vi "Simulate Rop Graph.vi"() -> ()   [LabVIEW 2020, in "AoC 2022.lvlib"]
uses:
  AoC 2022.lvlib
panel:
  in  "Puzzle Input":string="L 1\nD 2\nU 1\nL 1\nR 2\nL 2\nU 1\nD 2\nR 2\nL 2\nU 1\nD 2\nR 1\nD 2\nL 2\nD 1\nL 2\nR 1\nU 2\nR 2\nU 2\nL 2\nU 1\nL 2\nR 1\nD 1\nR 1\nL 1\nR 1\nL 1\nR 1\nU 1\nR 1\nL 1\nD 2\nL 2\nD 2\nL 1\nR 1\nD 1\nR 1\nD 2\nL 1\nD 2\nL 1\nR 2\nD 2\nR 2\nU 1\nR 1\nU 2\nR 1\nU 2\nR 1\nD 2\nL 1\nD 2\nU 1\nR 2\nD 2\nL 1\nU 2\nR 2\nL 2\nD 2\nL 2\nD 2\nR 1\nU 2\nL 2\nU 1\nR 1\nD 1\nL 1\nD 1\nU 1\nD 2\nL 1\nR 1\nD 1\nR 1\nL 2\nR 1\nL 1\nU 2\nD 2\nU 1\nL 1\nU 2\nR 1\nD 2\nU 1\nD 1\nL 1\nD 2\nU 2\nD 1\nU 2\nR 2\nL 2\nD 1\nR 2\nD 1\nL 2\nD 2\nL 2\nR 1\nL 1\nR 2\nL 2\nR 2\nU 1\nR 1\nU 3\nD 2\nU 3\nL 1\nR 1\nU 3\nD 1\nL 1\nR 3\nD 2\nL 3\nR 3\nD 2\nR 2\nU 3\nR 3\nU 3\nR 2\nU 3\nD 2\nL 3\nU 3\nR 1\nU 1\nR 3\nU 2\nL 1\nR 1\nU 1\nL 3\nR 3\nU 3\nD 2\nU 1\nL 1\nD 3\nR 3\nU 2\nL 1\nR 3\nL 3\nD 3\nU 3\nR 2\nL 1\nU 1\nL 3\nR 3\nU 1\nR 3\nL 2\nR 2\nD 3\nU 1\nD 3\nU 3\nR 3\nD 2\nL 2\nU 2\nD 3\nL 3\nU 3\nR 3\nD 2\nR 3\nU 1\nD 1\nU 2\nR 1\nD 3\nR 1\nL 2\nU 3\nD 1\nL 1\nD 3\nU 2\nL 3\nR 3\nL 1\nD 2\nL 3\nU 3\nL 1\nD 2\nL 1\nD 1\nL 2\nU 2\nD 2\nU 2\nL 2\nD 3\nL 3\nD 3\nR 3\nU 1\nR 3\nU 1\nR 3\nD 3\nU 2\nD 1\nR 2\nL 2\nR 2\nD 2\nR 2\nD 1\nR 3\nD 1\nU 2\nL 4\nD 1\nL 2\nR 1\nU 1\nD 3\nU 4\nD 2\nL 3\nR 2\nD 3\nR 4\nU 1\nD 1\nU 1\nL 3\nU 1\nD 3\nR 3\nD 3\nR 1\nU 4\nR 1\nU 1\nR 2\nL 4\nU 3\nD 2\nR 2\nD 1\nU 2\nL 3\nD 4\nU 4\nD 4\nU 4\nL 3\nU 3\nD 3\nR 3\nL 4\nR 3\nD 2\nL 2\nR 1\nD 1\nL 4\nR 3\nD 2\nU 1\nL 2\nR 1\nU 2\nL 4\nR 4\nL 3\nU 4\nD 2\nU 4\nD 4\nL 1\nU 4\nL 3\nU 2\nD 2\nR 2\nD 3\nR 4\nD 1\nU 4\nD 1\nU 1\nD 3\nL 3\nD 2\nR 4\nD 4\nL 2\nU 2\nL 3\nR 4\nL 2\nR 2\nD 3\nL 2\nD 4\nU 3\nD 4\nL 3\nR 2\nU 3\nD 4\nR 2\nU 3\nR 1\nD 1\nR 1\nD 2\nR 3\nD 4\nL 1\nU 3\nL 3\nU 4\nR 1\nU 3\nL 4\nD 5\nR 2\nD 2\nU 2\nD 1\nR 4\nD 1\nL 4\nD 4\nL 1\nR 1\nD 4\nU 4\nL 1\nD 4\nL 4\nU 5\nR 4\nD 4\nR 5\nU 3\nL 5\nU 1\nR 4\nL 1\nR 3\nL 2\nD 5\nR 1\nD 4\nR 2\nU 5\nL 3\nR 5\nU 4\nR 1\nD 4\nU 3\nR 3\nL 3\nR 3\nL 3\nU 2\nD 4\nU 2\nL 3\nD 2\nR 3\nU 3\nD 2\nU 1\nR 5\nL 4\nR 4\nL 4\nD 3\nR 3\nU 2\nR 1\nD 3\nU 3\nD 2\nL 1\nD 2\nU 1\nL 3\nU 5\nL 1\nD 1\nU 5\nD 3\nU 4\nD 4\nL 5\nR 3\nD 4\nR 2\nL 1\nD 1\nL 3\nU 3\nR 1\nL 2\nD 4\nL 5\nU 1\nL 4\nR 4\nU 2\nD 1\nR 5\nD 3\nU 2\nD 3\nU 4\nD 4\nU 1\nL 2\nD 4\nL 3\nU 4\nL 1\nR 1\nL 2\nR 3\nL 2\nU 1\nD 2\nU 5\nR 2\nD 4\nU 1\nD 4\nU 4\nD 5\nL 6\nD 3\nU 2\nD 1\nL 3\nU 4\nR 4\nD 4\nR 3\nL 4\nU 6\nD 1\nU 4\nR 2\nL 1\nD 2\nU 4\nD 5\nU 3\nD 6\nL 1\nU 3\nL 1\nU 1\nD 6\nL 3\nU 6\nL 3\nD 6\nL 1\nD 6\nU 2\nD 5\nU 2\nL 5\nD 3\nU 2\nD 1\nU 6\nL 1\nD 4\nL 6\nR 3\nD 3\nL 3\nD 2\nR 3\nD 5\nR 3\nD 2\nL 1\nR 4\nL 6\nD 4\nR 4\nU 1\nR 6\nD 3\nU 1\nR 1\nD 1\nL 3\nD 1\nR 3\nU 5\nL 5\nD 2\nL 3\nD 2\nL 5\nU 3\nL 1\nU 5\nL 3\nD 4\nU 5\nD 1\nL 6\nD 1\nR 6\nU 4\nR 1\nD 1\nL 2\nU 5\nR 2\nU 6\nL 5\nU 5\nL 6\nU 6\nD 3\nL 1\nR 3\nL 3\nU 4\nR 5\nL 6\nD 5\nL 4\nR 6\nL 6\nR 5\nD 2\nR 4\nL 2\nU 1\nL 3\nU 6\nL 4\nD 6\nU 6\nD 4\nL 2\nR 7\nU 4\nR 1\nL 5\nD 2\nR 3\nU 4\nL 5\nU 7\nL 2\nR 1\nU 4\nL 2\nR 5\nL 6\nD 5\nL 4\nU 5\nL 7\nU 1\nL 5\nU 1\nL 5\nD 3\nU 3\nR 7\nU 7\nR 7\nL 6\nD 4\nU 7\nR 2\nD 3\nR 3\nU 4\nD 4\nU 5\nD 6\nL 5\nR 6\nU 4\nR 6\nD 1\nR 4\nU 1\nD 1\nR 1\nL 4\nU 5\nL 3\nD 5\nL 5\nD 3\nU 2\nR 5\nD 7\nU 7\nD 1\nU 5\nR 6\nU 4\nR 6\nL 7\nU 5\nR 1\nL 1\nU 1\nR 1\nD 7\nL 2\nU 5\nR 4\nU 2\nD 6\nU 6\nL 7\nU 3\nD 2\nL 3\nR 3\nU 2\nL 1\nR 2\nL 5\nD 6\nR 2\nU 6\nL 1\nD 7\nR 4\nD 3\nL 2\nU 5\nR 4\nL 2\nR 5\nD 1\nU 1\nR 6\nD 5\nU 6\nR 2\nU 2\nL 2\nU 6\nL 5\nU 1\nL 1\nD 7\nR 6\nU 5\nD 3\nL 5\nR 3\nD 3\nU 2\nD 7\nU 7\nL 1\nD 5\nL 5\nU 4\nL 5\nD 1\nU 6\nD 5\nL 7\nD 8\nU 8\nR 6\nU 5\nD 8\nU 1\nR 2\nU 6\nD 6\nL 4\nD 2\nR 3\nU 7\nR 4\nU 4\nR 5\nU 6\nR 1\nU 4\nR 1\nU 4\nD 5\nU 3\nL 7\nU 8\nR 1\nD 1\nU 8\nL 8\nU 3\nL 1\nD 4\nR 2\nD 4\nU 2\nL 4\nD 8\nR 7\nD 5\nU 4\nL 5\nU 5\nD 8\nR 8\nU 3\nR 8\nL 4\nU 5\nR 6\nU 7\nD 3\nL 1\nU 5\nD 2\nR 5\nU 4\nD 8\nL 4\nR 1\nD 6\nR 1\nL 6\nD 6\nL 7\nD 4\nL 4\nD 8\nR 8\nD 7\nL 6\nR 1\nD 4\nL 5\nD 2\nU 3\nD 2\nU 6\nR 1\nU 7\nD 7\nR 2\nU 7\nD 5\nL 6\nU 1\nL 8\nU 1\nL 1\nR 9\nD 1\nU 6\nD 5\nL 1\nR 9\nD 2\nL 2\nD 6\nU 6\nD 7\nL 3\nR 5\nL 6\nU 5\nR 1\nU 1\nR 3\nL 9\nU 6\nL 6\nU 2\nD 6\nR 9\nU 4\nD 3\nL 8\nU 5\nD 7\nL 1\nU 7\nR 1\nL 6\nD 8\nL 5\nR 7\nL 2\nR 6\nL 5\nD 3\nL 8\nD 7\nU 8\nR 6\nL 6\nD 7\nU 8\nD 1\nU 2\nD 5\nU 7\nD 8\nL 1\nD 1\nL 1\nU 1\nR 3\nL 5\nR 9\nD 2\nL 8\nR 6\nD 6\nU 1\nR 7\nL 4\nU 4\nD 1\nL 5\nU 2\nR 9\nD 7\nU 8\nL 8\nR 4\nD 1\nL 1\nU 7\nR 8\nL 3\nD 2\nU 8\nR 1\nD 5\nL 1\nR 7\nD 6\nR 2\nU 9\nD 2\nL 5\nU 4\nD 9\nL 7\nD 9\nL 2\nU 9\nD 5\nL 7\nD 6\nU 5\nD 9\nR 3\nU 8\nL 7\nU 1\nL 3\nU 3\nD 1\nL 6\nR 9\nU 2\nL 7\nR 9\nU 5\nR 2\nL 3\nR 4\nD 9\nL 4\nR 9\nU 4\nL 10\nR 9\nD 9\nU 10\nL 2\nR 4\nU 4\nR 9\nD 2\nR 1\nL 4\nR 7\nD 3\nL 6\nU 1\nL 9\nD 6\nU 10\nD 1\nR 10\nD 9\nL 6\nD 10\nU 3\nR 10\nL 8\nU 9\nD 1\nL 1\nD 10\nL 1\nD 5\nL 9\nU 3\nL 4\nU 4\nD 1\nU 3\nR 7\nL 3\nR 3\nL 3\nR 8\nD 9\nR 4\nL 6\nD 7\nR 10\nU 6\nR 2\nD 2\nL 3\nR 9\nD 9\nU 7\nD 2\nR 6\nU 10\nR 8\nU 5\nR 5\nU 10\nR 6\nU 7\nL 7\nU 7\nD 4\nL 9\nU 2\nR 7\nL 8\nR 4\nL 1\nU 9\nR 8\nD 4\nR 5\nD 4\nL 1\nD 10\nR 8\nD 10\nU 9\nD 3\nR 1\nU 10\nR 1\nD 10\nR 1\nL 6\nD 3\nU 8\nR 4\nU 9\nD 8\nU 3\nD 2\nR 3\nL 5\nU 4\nL 3\nR 4\nD 6\nL 9\nR 1\nD 9\nR 2\nD 11\nR 8\nD 5\nR 8\nL 2\nD 2\nL 7\nU 11\nD 10\nL 6\nR 2\nU 9\nL 10\nD 4\nL 5\nR 7\nD 4\nL 1\nU 3\nL 9\nD 7\nR 4\nD 10\nL 5\nU 9\nL 10\nD 5\nL 11\nR 11\nU 8\nR 11\nU 2\nR 7\nL 10\nR 2\nD 8\nL 2\nD 8\nR 11\nL 6\nR 3\nL 2\nU 2\nR 2\nU 3\nD 3\nU 5\nL 8\nU 9\nR 10\nD 1\nU 4\nD 8\nR 3\nD 11\nR 4\nD 4\nR 7\nU 6\nL 11\nU 11\nD 8\nL 5\nR 2\nL 11\nU 7\nD 5\nU 5\nD 9\nL 2\nU 3\nR 10\nU 1\nR 1\nL 11\nD 3\nL 5\nR 2\nL 10\nR 4\nL 1\nU 1\nL 4\nR 5\nU 2\nD 6\nR 11\nU 8\nD 5\nR 5\nD 3\nL 2\nU 7\nD 10\nL 11\nD 10\nU 11\nR 8\nL 2\nD 9\nR 9\nL 11\nR 10\nU 3\nR 4\nL 5\nR 12\nU 5\nD 5\nL 6\nD 11\nR 8\nD 12\nU 6\nL 10\nR 9\nU 1\nL 12\nD 1\nR 8\nU 9\nD 9\nR 6\nD 3\nL 1\nR 3\nL 8\nR 6\nU 12\nL 1\nU 8\nD 7\nU 5\nD 12\nL 4\nR 11\nU 9\nD 12\nR 8\nD 2\nR 7\nU 8\nR 10\nU 3\nR 4\nD 4\nU 9\nR 7\nL 9\nR 7\nU 8\nL 9\nU 6\nR 4\nL 11\nD 11\nR 6\nU 2\nD 1\nR 2\nL 2\nD 11\nR 5\nU 1\nR 1\nD 3\nU 2\nL 3\nU 12\nR 10\nU 12\nR 9\nD 11\nU 9\nL 2\nR 7\nU 5\nR 7\nU 9\nR 3\nD 4\nL 9\nD 4\nR 12\nL 3\nU 12\nL 9\nU 3\nL 11\nR 7\nU 11\nD 2\nL 11\nR 2\nL 12\nU 10\nL 6\nR 8\nD 6\nR 12\nL 7\nR 4\nU 5\nD 10\nR 8\nL 11\nD 4\nU 1\nR 9\nU 12\nD 3\nL 10\nR 11\nU 1\nL 5\nU 11\nL 7\nU 1\nD 13\nU 10\nL 12\nU 9\nD 8\nL 5\nR 4\nL 1\nR 2\nL 7\nD 1\nL 11\nU 9\nR 5\nD 12\nL 4\nU 7\nL 6\nR 7\nU 1\nL 7\nU 2\nD 4\nR 4\nD 7\nL 3\nD 9\nU 3\nD 3\nU 12\nR 2\nL 12\nR 9\nL 8\nD 10\nU 1\nR 11\nL 13\nU 1\nD 3\nU 12\nL 3\nR 7\nL 7\nD 7\nU 7\nD 7\nU 10\nD 1\nL 7\nD 11\nR 3\nD 6\nR 9\nD 5\nU 12\nD 6\nR 8\nD 3\nR 7\nL 6\nD 10\nU 8\nR 9\nD 4\nR 9\nD 2\nU 4\nR 4\nU 7\nL 12\nR 2\nD 10\nU 13\nR 12\nL 12\nD 1\nR 11\nL 2\nU 13\nL 12\nD 7\nL 2\nU 4\nL 4\nD 8\nL 9\nR 3\nD 4\nL 9\nU 9\nL 9\nR 10\nL 4\nR 4\nU 10\nL 11\nD 8\nU 8\nL 13\nR 1\nL 8\nU 13\nL 9\nU 1\nR 13\nU 7\nL 3\nR 8\nL 1\nD 5\nR 7\nU 8\nD 5\nL 12\nR 11\nU 11\nD 10\nU 5\nR 6\nD 11\nR 1\nD 1\nR 9\nL 8\nD 4\nL 11\nU 9\nD 4\nU 3\nD 13\nU 13\nL 6\nD 6\nR 11\nL 9\nU 3\nR 7\nD 9\nR 5\nL 9\nD 14\nR 8\nL 14\nR 6\nL 6\nU 6\nR 7\nL 11\nR 1\nL 6\nD 10\nR 1\nD 14\nR 12\nU 4\nR 2\nL 9\nR 14\nL 3\nD 9\nU 10\nR 11\nL 5\nR 14\nU 3\nD 8\nR 9\nL 13\nU 4\nL 2\nR 4\nD 6\nL 13\nD 4\nR 2\nL 2\nD 10\nL 10\nR 4\nD 2\nR 2\nU 6\nD 7\nU 12\nR 5\nU 13\nL 6\nU 12\nL 3\nD 11\nR 3\nL 7\nU 11\nD 4\nL 13\nU 14\nR 10\nD 12\nU 2\nL 1\nU 12\nD 6\nU 2\nR 12\nL 3\nD 9\nU 9\nR 14\nL 12\nR 5\nL 11\nR 11\nL 5\nR 2\nL 4\nD 8\nU 3\nR 4\nD 12\nR 10\nL 10\nD 10\nU 10\nR 9\nL 14\nR 3\nL 1\nD 1\nR 15\nD 15\nR 12\nL 15\nD 12\nL 10\nR 3\nU 14\nD 4\nU 7\nR 11\nL 10\nU 4\nD 15\nL 3\nU 1\nR 2\nL 15\nU 6\nL 6\nD 3\nL 14\nD 12\nU 1\nL 15\nR 13\nU 7\nD 6\nR 11\nU 7\nL 2\nD 11\nL 1\nR 7\nD 1\nL 4\nR 11\nU 5\nL 4\nR 13\nU 1\nD 4\nL 6\nR 10\nL 15\nU 7\nD 9\nL 10\nR 8\nU 10\nD 8\nL 14\nD 15\nR 14\nU 10\nD 4\nU 6\nD 2\nR 6\nL 6\nD 4\nU 12\nL 3\nR 6\nU 9\nR 3\nU 11\nR 3\nU 15\nD 1\nU 2\nD 3\nU 11\nL 3\nU 2\nL 14\nD 3\nR 9\nD 5\nL 10\nU 7\nL 6\nD 8\nL 8\nU 8\nL 14\nR 9\nL 14\nU 10\nL 8\nU 5\nL 2\nU 4\nD 5\nR 2\nL 1\nU 14\nR 3\nL 4\nU 9\nD 7\nU 14\nD 11\nR 9\nU 5\nR 8\nL 5\nU 3\nD 8\nR 8\nL 11\nR 7\nL 3\nD 16\nL 11\nU 7\nD 6\nR 5\nL 4\nU 9\nL 12\nR 9\nL 10\nD 13\nL 3\nD 13\nU 6\nR 14\nU 2\nL 5\nR 4\nL 15\nU 9\nD 5\nL 6\nR 7\nU 10\nL 3\nD 5\nU 8\nD 12\nL 11\nU 14\nD 12\nU 2\nD 9\nU 11\nD 5\nL 5\nR 10\nL 14\nU 1\nR 8\nD 5\nR 6\nU 6\nL 3\nU 11\nL 8\nR 3\nU 5\nL 1\nR 16\nD 10\nU 12\nR 11\nD 2\nU 4\nD 15\nU 16\nD 2\nL 9\nR 10\nL 3\nU 8\nR 13\nU 11\nD 12\nU 15\nD 1\nL 14\nR 3\nU 13\nD 7\nR 15\nL 3\nR 1\nU 7\nR 6\nD 12\nL 2\nR 13\nD 3\nR 6\nD 10\nU 2\nR 4\nD 12\nL 7\nR 7\nL 8\nR 14\nL 15\nD 8\nL 6\nU 14\nL 16\nU 10\nD 7\nR 6\nD 12\nR 16\nU 11\nR 2\nU 10\nL 1\nR 6\nU 14\nD 13\nU 7\nL 10\nD 4\nL 7\nR 11\nU 17\nD 6\nU 6\nR 6\nU 12\nL 16\nU 5\nR 15\nL 17\nD 13\nU 12\nL 1\nD 7\nL 13\nR 7\nU 2\nL 5\nU 12\nR 10\nU 7\nR 11\nU 17\nD 15\nU 15\nL 10\nD 3\nL 15\nU 8\nR 8\nD 10\nL 9\nU 6\nR 9\nL 1\nU 5\nR 6\nL 11\nD 17\nL 7\nU 3\nD 17\nR 17\nU 8\nL 15\nR 3\nD 2\nU 17\nL 1\nR 13\nU 13\nL 10\nR 2\nD 12\nL 12\nR 13\nL 14\nR 16\nD 12\nR 4\nU 14\nL 15\nR 10\nD 7\nR 12\nU 6\nL 8\nU 7\nR 1\nD 3\nR 3\nL 11\nD 2\nR 15\nU 17\nL 13\nU 17\nD 4\nU 11\nL 17\nD 12\nR 3\nL 12\nU 8\nD 2\nL 14\nU 16\nD 6\nU 7\nL 12\nR 17\nL 7\nD 1\nL 16\nD 16\nR 17\nD 5\nU 16\nD 2\nL 13\nU 9\nD 13\nR 3\nU 1\nD 12\nR 4\nD 11\nL 8\nD 8\nR 13\nD 16\nR 1\nD 10\nR 18\nU 6\nD 4\nU 17\nR 12\nL 14\nU 5\nL 15\nU 18\nR 4\nD 17\nL 4\nR 18\nU 18\nD 4\nL 1\nU 4\nL 2\nU 17\nR 16\nL 7\nU 10\nR 11\nU 9\nR 11\nL 16\nU 3\nR 3\nL 18\nU 8\nR 1\nU 1\nL 5\nU 5\nD 7\nL 1\nR 2\nU 16\nR 17\nD 4\nU 16\nL 12\nR 3\nL 16\nD 5\nU 5\nR 18\nL 7\nU 1\nL 7\nU 16\nR 14\nL 4\nR 13\nL 3\nU 4\nL 11\nU 3\nL 12\nU 16\nL 14\nU 3\nL 9\nR 18\nD 8\nL 15\nR 10\nD 2\nL 13\nD 11\nU 4\nL 13\nD 7\nL 12\nU 7\nD 17\nU 9\nD 5\nL 10\nR 2\nD 7\nL 14\nU 10\nD 17\nL 3\nR 17\nU 16\nD 13\nR 13\nU 14\nR 9\nL 3\nU 14\nL 7\nU 4\nD 1\nR 18\nU 11\nD 9\nU 8\nR 15\nL 5\nD 9\nL 2\nD 18\nU 12\nD 3\nU 14\nD 9\nU 13\nR 16\nU 8\nR 16\nU 4\nL 8\nD 14\nR 15\nD 6\nR 17\nU 6\nD 1\nL 2\nU 9\nD 15\nL 7\nD 3\nR 1\nL 1\nR 17\nD 12\nR 19\nU 4\nR 19\nL 2\nD 17\nU 11\nD 1\nL 9\nR 18\nL 7\nD 13\nU 6\nD 16\nL 6\nR 13\nU 12\nR 1\nL 2\nU 8\nL 16\nR 10\nD 15\nR 5\nL 1\nU 5\nR 18\nU 1\nR 4\nU 14\nR 3\nL 4\nU 13\nD 14\nL 10\nD 7\nU 3\nR 17\nL 19\nR 1\nD 12\nL 9\nU 19\nD 19\nL 5\nR 10\nL 14\nU 15\nD 19\nU 18\nD 14\nR 11\nU 8\nR 2\nU 16\nL 17\nD 6\nL 1\nD 10\nR 18\nU 5\nR 14\nU 10\nD 6\nL 17\nD 6\nU 7\nR 14\nL 1\nU 3\nD 3\nR 18\nD 1\nL 6\nD 18\nL 2\nR 10\nL 9\nR 10\nL 14\nR 15\nU 10"
  in  "Use Buggy Movement?":bool
  in  "#Knots":i32=10 max=11517
  in  "Load Input":bool
  out "Grid":string
  in  "Step":i32(slide) caption="U" max=11517 scale=0.0..11517.0
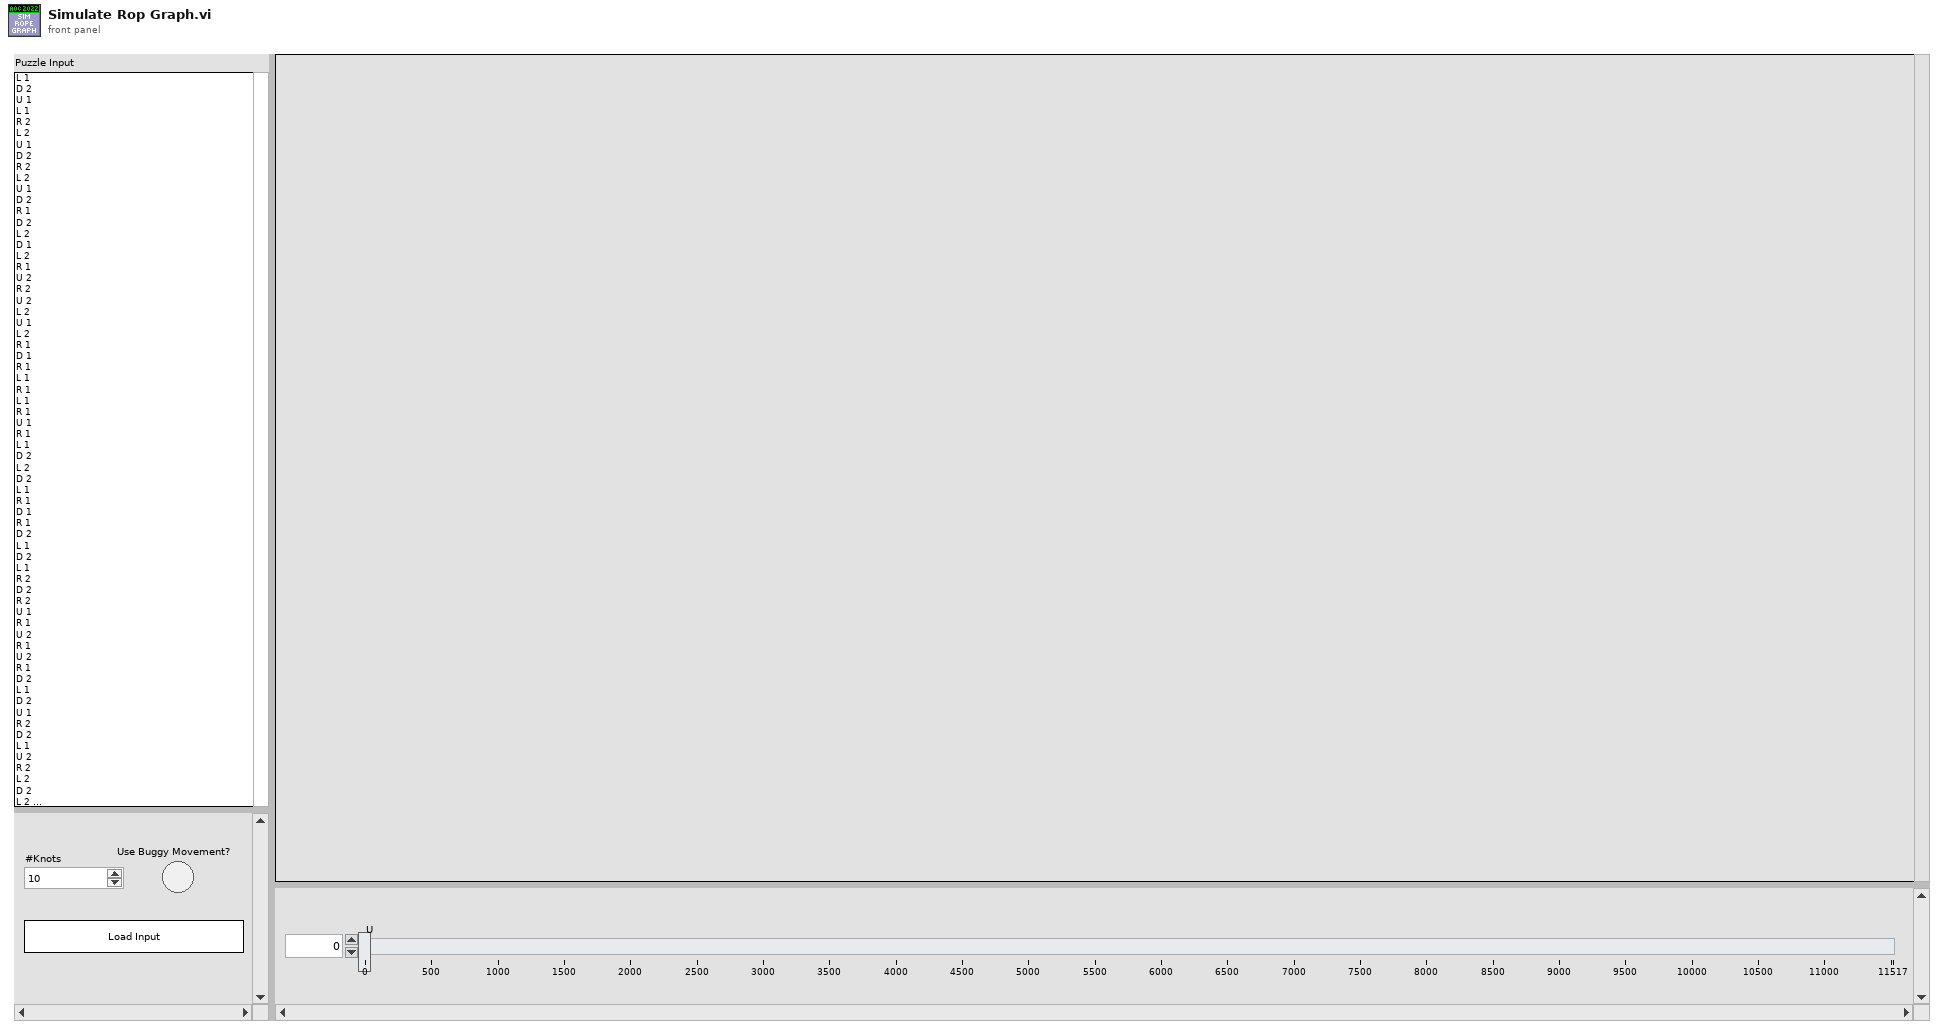
[diagram p1: front panel]
types:
  T1 = typedef "AoC 2022.lvlib/Rope Data.ctl" = map{i32, T2}
  T2 = typedef "AoC 2022.lvlib/Positions.ctl" = cluster{"H Direction":string, "H":cdb, "Knots":cdb[], "T":cdb}
  T3 = cluster{"Rope Data":T1, "Rows":i32, "Columns":i32, "Offset":cdb}
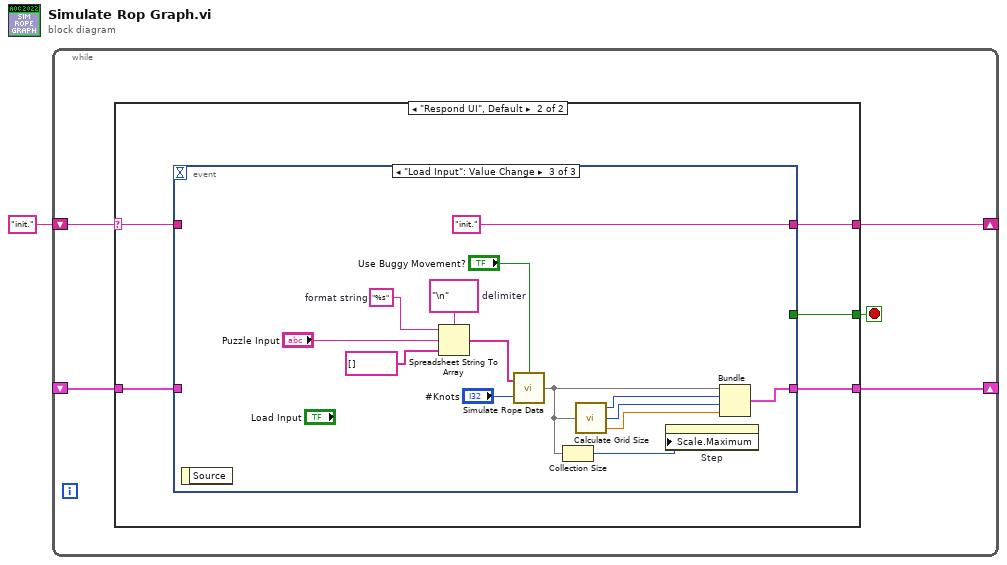
[diagram p0: block diagram]
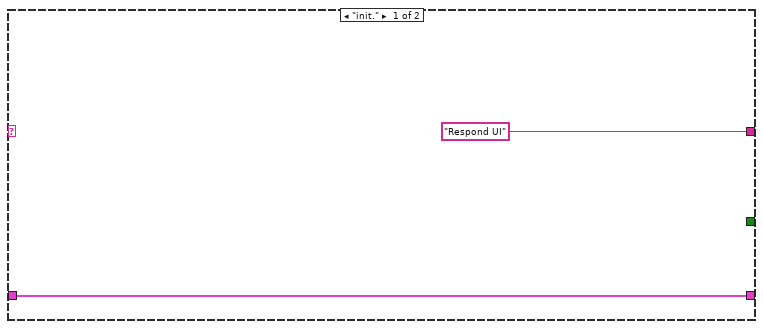
[diagram p2: hidden frame]
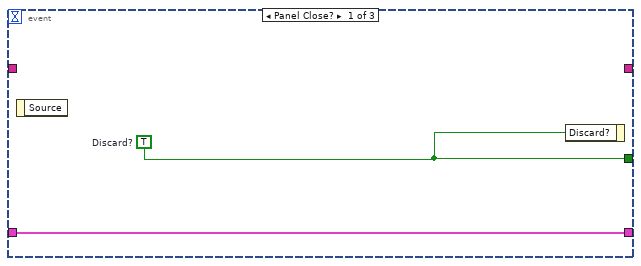
[diagram p3: hidden frame]
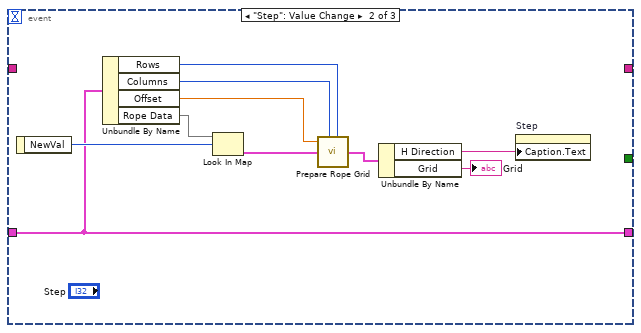
[diagram p4: hidden frame]
diagram:
  n1 = while {
    shift-right: [w4] -> _
    shift-left: "init." -> [w5]
    shift-right: [w3] -> _
    shift-left: _ -> [w2]
    stop <- w6 stop-if-true
    n2 = case shown="\"Respond UI\", Default" w5 {
      selector: w5 -> [_ w12]
      tunnel: [_ w13] -> w6
      tunnel: ["Respond UI" w11] -> w4
      tunnel: [w7 w10] -> w3
      tunnel: w2 -> [w7 w9]
      frame "init." {
      }
      frame "Respond UI", Default {
        n3 = event shown="[2] \"Load Input\": Value Change" {
          selector: _ -> [_ _ _]
          dyn-events: _ -> [_ _ _]
          timeout: _ -> [_ _ _]
          tunnel: [w15 _ _] -> w13
          tunnel: w12 -> [_ _ _]
          tunnel: [_ _ "init."] -> w11
          tunnel: [w14 w23 w32] -> w10
          tunnel: w9 -> [w14 w23 _]
          event Panel Close? {
            w15 = TRUE  # Discard?
            n4 = event-data() -> ()  [unwired: 1 in, 1 out]
            n5 = event-data("Discard?"=w15) -> ()  [unwired: 1 in, 1 out]
          }
          event "Step": Value Change {
            n6 = event-data() -> ("NewVal"=w25:i32)  [unwired: 1 in]
            n7 = Unbundle By Name(w23) -> ("Rows"=w21:i32, "Columns"=w20:i32, "Offset"=w16:cdb, "Rope Data"=w22:T1)
            n8 = Look In Map(map=w22, key=w25) -> (value=w17:T2)  [unwired: 1 in, 1 out]
            n9 = call "Prepare Rope Grid.vi"("Offset"=w16, "Columns"=w20, "Positions"=w17, "Rows"=w21) -> ("Rope Grid"=w24:cluster{"Grid":string, "H Direction":string})  [unwired: 4 in, 1 out]
            n10 = Unbundle By Name(w24) -> ("H Direction"=w19:string, "Grid"=→"Grid":string)
            n11 = property on="Step" class="Slide (strict)"("Caption.Text"=w19) -> ()  [unwired: 2 in, 2 out]
          }
          event "Load Input": Value Change {
            w36 = "%s"  # format string
            w38 = "\n"  # delimiter
            n12 = event-data() -> ()  [unwired: 1 in, 1 out]
            n13 = Spreadsheet String To Array(delimiter (Tab)=w38, format string=w36, spreadsheet string="Puzzle Input", array type (2D Dbl)=string[] []) -> (array=w34:string[])
            n14 = call "Simulate Rope Data.vi"("Use Buggy Movement?"="Use Buggy Movement?", "#Knots"="#Knots", "Moves"=w34) -> ("Rope Data"=w28:T1)
            n15 = Collection Size(1:w28) -> (0:w27:i32)
            n16 = call "Calculate Grid Size.vi"("Rope Data"=w28) -> ("Rows"=w30:i32, "Columns"=w29:i32, "Offset"=w31:cdb)
            n17 = property on="Step" class="Slide (strict)"("Scale.Maximum"=w27) -> ()  [unwired: 2 in, 2 out]
            n18 = Bundle("Rope Data"=w28, "Rows"=w30, "Columns"=w29, "Offset"=w31) -> (w32:T3)  [unwired: 1 in]
          }
        }
      }
    }
  }
